vi "Write TCPQueueName.vi"(8 "error in (no error)":errorcluster, 10 "TCPQueueName":string, 11 "Server in":refnum<class "Server.lvclass">) -> (0 "error out":errorcluster, 3 "Server out":refnum<class "Server.lvclass">)   [LabVIEW 2018, in "Server.lvclass"]
uses:
  Server.lvclass
  Server.lvclass/Server.ctl
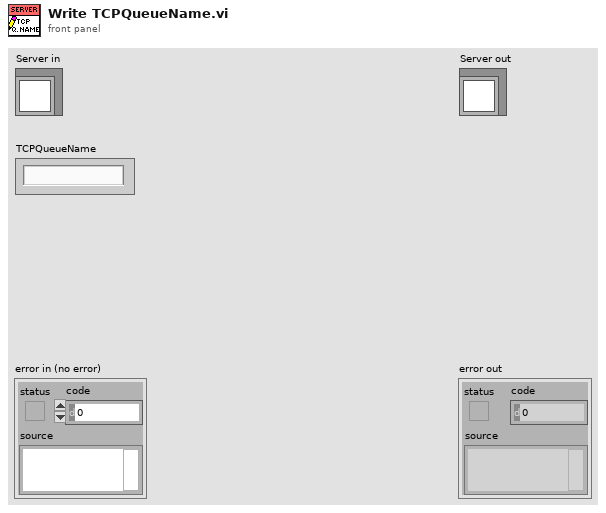
[diagram p1: front panel]
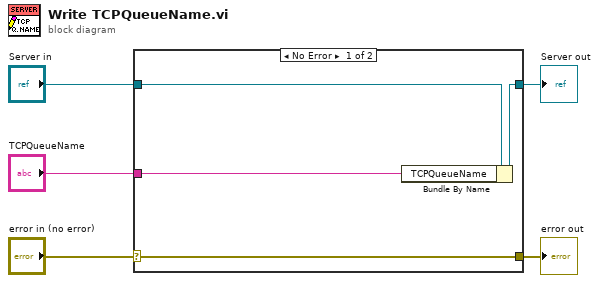
[diagram p0: block diagram]
diagram:
  n1 = case shown="No Error" "error in (no error)" {
    selector: "error in (no error)" -> [w9 w10]
    tunnel: [w9 w10] -> w4
    tunnel: [w7 w11] -> w2
    tunnel: "Server in" -> [w8 w11]
    tunnel: "TCPQueueName" -> [w6 _]
    frame No Error {
      n2 = Bundle By Name(cluster=w8, "TCPQueueName"=w6) -> (w7:refnum<class "Server.lvclass">)
    }
    frame Error {
    }
  }
  "error out" <- w4
  "Server out" <- w2
